vi "DAC RH FP Conf.vi"(8 "error in":errorcluster, 9 "RH Active":bool, 10 "Result Unit":string, 11 "DeepU Results in":refnum<class "DeepU Results.lvclass">) -> (0 "error out":errorcluster, 3 "DeepU Results out":refnum<class "DeepU Results.lvclass">)   [LabVIEW 2019, in "Results.lvlib" / "DeepU Results.lvclass"]
uses:
  DeepU Results.lvclass
  DeepU Results.lvclass/DeepU Results.ctl
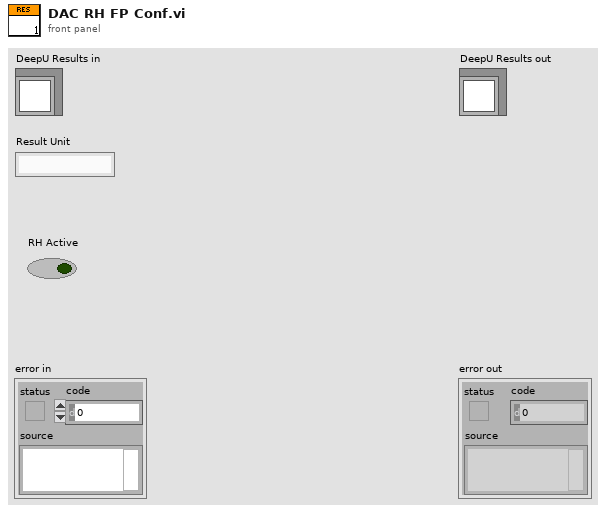
[diagram p1: front panel]
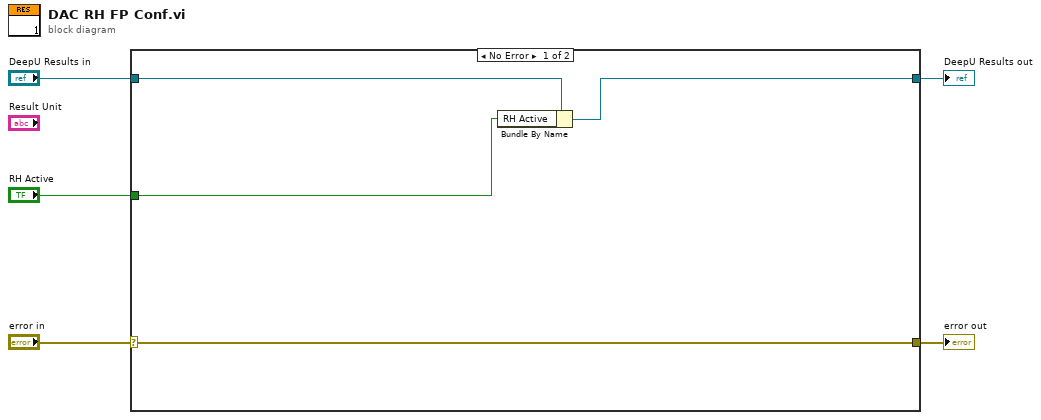
[diagram p0: block diagram]
diagram:
  n1 = case shown="No Error" "error in" {
    selector: "error in" -> [w9 w11]
    tunnel: [w9 w11] -> w4
    tunnel: [w7 w10] -> w2
    tunnel: "DeepU Results in" -> [w8 w10]
    tunnel: "RH Active" -> [w6 _]
    frame No Error {
      n2 = Bundle By Name(cluster=w8, "RH Active"=w6) -> (w7:refnum<class "DeepU Results.lvclass">)
    }
    frame Error {
    }
  }
  "error out" <- w4
  "DeepU Results out" <- w2
